vi "Buzzer.vi"(8 "error in (no error)":errorcluster, 10 "Buzzer (0:Buzzer On)":enum16{"Buzzer On", "Buzzer Off"}(ring), 11 "VISA resource name":refnum<visa-resource-name>) -> (0 "error out":errorcluster, 3 "VISA resource name out":refnum<visa-resource-name>)   [LabVIEW 2021, in "Siglent SDS 1000 2000 Series.lvlib"]
doc: "Configures the system buzzer."
uses:
  <instrlib>/Siglent SDS 1000 2000 Series/Siglent SDS 1000 2000 Series.lvlib
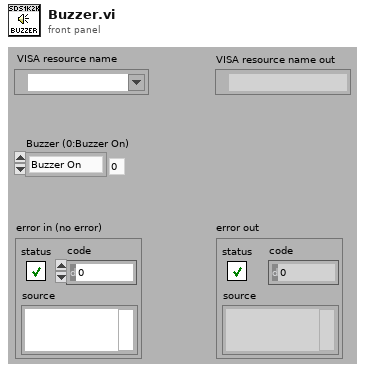
[diagram p1: front panel]
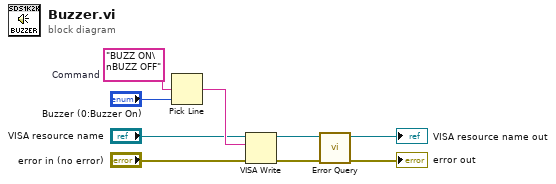
[diagram p0: block diagram]
diagram:
  w7 = "BUZZ ON\nBUZZ OFF"  # Command
  n1 = Pick Line(multi-line string=w7, line index="Buzzer (0:Buzzer On)") -> (output string=w6:string)  [unwired: 1 in]
  n2 = VISA Write(VISA resource name="VISA resource name", write buffer=w6, error in (no error)="error in (no error)") -> (VISA resource name out=w2:refnum<visa-resource-name>, error out=w1:errorcluster)  [unwired: 1 out]
  n3 = call <instrlib>:"Error Query.vi"("error in (no error)"=w1, "VISA resource name"=w2) -> ("error out"=→"error out":errorcluster, "VISA resource name out"=→"VISA resource name out":refnum<visa-resource-name>)  [unwired: 6 in, 2 out]
